vi "Begin.vi"(8 "error in":errorcluster) -> (0 "error out":errorcluster)   [LabVIEW 2016]
doc: "Called before other user functions, this VI is expected to open initial I/O refnums, load in file data, and do all program initialization. Notice that the <B>error out</B> terminal is simply used for data flow. Wiring it to other structures or subVIs ensures that this VI runs first."
uses:
  <vilib>/Rock Robotics/WPI/DriverStation/WPI_DriverStationRobotMode2.ctl
  Control Files/DriveMotors.ctl
  Control Files/Extra Motors.ctl
  <vilib>/Rock Robotics/WPI/ThirdParty/CanMotor/TalonSRX/WPI_CANTalonSRX_APIControlMode.ctl
  Control Files/Controllers.ctl
  <vilib>/Rock Robotics/WPI/Joystick/WPI_JoystickDeviceEnum.ctl
  <vilib>/Rock Robotics/WPI/SafetyOutput/WPI_SafetyOutputConfigMenu.ctl
  Control Files/SwerveMotors.ctl
  <vilib>/Rock Robotics/WPI/ThirdParty/CanMotor/TalonSRX/WPI_CANTalonSRX_APIFeedbackSelect.ctl
  Robot Global Data.vi
panel:
  in  "PID gains":T1={"proportional gain (Kc)"=5.0, "integral time (Ti, min)"=0.032, "derivative time (Td, min)"=0.0} {"derivative time (Td, min)" format="%.3f"; "integral time (Ti, min)" format="%.8f"; "proportional gain (Kc)" format="%.8f"}
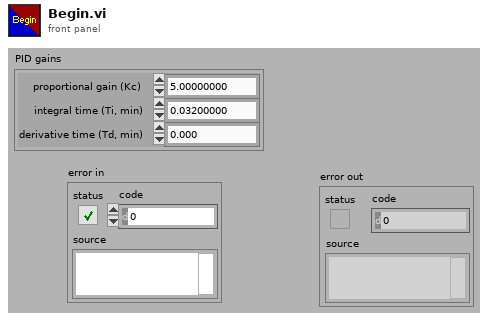
[diagram p1: front panel]
types:
  T1 = cluster{"proportional gain (Kc)":dbl, "integral time (Ti, min)":dbl, "derivative time (Td, min)":dbl}
  T2 = typedef "WPI_SafetyOutputConfigMenu.ctl" = enum16{"Enable", "Disable"}
  T3 = typedef "WPI_JoystickDeviceEnum.ctl" = enum16{"USB 0", "USB 1", "USB 2", "USB 3", "USB 4", "USB 5"}
  T4 = typedef "Controllers.ctl" = enum16{"Controller", "Controller2"}
  T5 = typedef "WPI_CANTalonSRX_APIControlMode.ctl" = enum8{"Percent VBus", "Speed", "Position", "Slave", "Unchanged / Invalid", "Voltage Compensation", "Current", "Motion Profile", "Motion Magic"}
  T6 = typedef "Extra Motors.ctl" = enum16{"Climber"}
  T7 = typedef "DriveMotors.ctl" = enum16{"Drive1", "Drive2", "Drive3", "Drive4"}
  T8 = typedef "WPI_DriverStationRobotMode2.ctl" = enum16{"Autonomous Disabled", "Autonomous Enabled", "Teleop Disabled", "Teleop Enabled", "Disconnected", "Finish", "Test Disabled", "Test Enabled", "Emergency Stopped"}
  T9 = typedef "WPI_CANTalonSRX_APIFeedbackSelect.ctl" = enum16{"Digital Quadrature Encoder", "Analog Potentiometer", "Analog Encoder", "Count on Quad-A (Rising-Edge)", "Count on Quad-A (Falling-Edge)", "CTR Magnetic Enc (Absolute)", "CTR Magnetic Enc (Relative)", "Pulse Width"}
  T10 = typedef "SwerveMotors.ctl" = enum16{"Swerve 1", "Swerve 2", "Swerve 3", "Swerve 4"}
  T11 = typedef "WPI_MotorControlDeviceRef.ctl" = cluster{"DeviceStatus":errorcluster, "Type":T12, "PWM":cluster{"PWM Channel":T13, "DeadBand":T14}, "CAN":cluster{"Device Number":u8, "SetOutput VI Ref":variant, "GetOutput VI Ref":variant, "Enable VI Ref":variant, "Disable VI Ref":variant, "Data":variant}, "Invert":bool}
  T12 = typedef "WPI_MotorControlType.ctl" = enum16{"PWM", "CAN"}
  T13 = typedef "FPGA_DIOPWMChannel.ctl" = enum8{"PWM 0", "PWM 1", "PWM 2", "PWM 3", "PWM 4", "PWM 5", "PWM 6", "PWM 7", "PWM 8", "PWM 9", "PWM MXP 0", "PWM MXP 1", "PWM MXP 2", "PWM MXP 3", "PWM MXP 4", "PWM MXP 5", "PWM MXP 6", "PWM MXP 7", "PWM MXP 8", "PWM MXP 9", "Invalid"}
  T14 = typedef "WPI_PWMDeadband.ctl" = cluster{"Name":string, "maxPositivePwm":i32, "minPositivePwm":i32, "centerPwm":i32, "maxNegativePwm":i32, "minNegativePwm":i32, "angularRange":u16}
  T15 = typedef "WPI_JoystickDevRef.ctl" = cluster{"Device":T3}
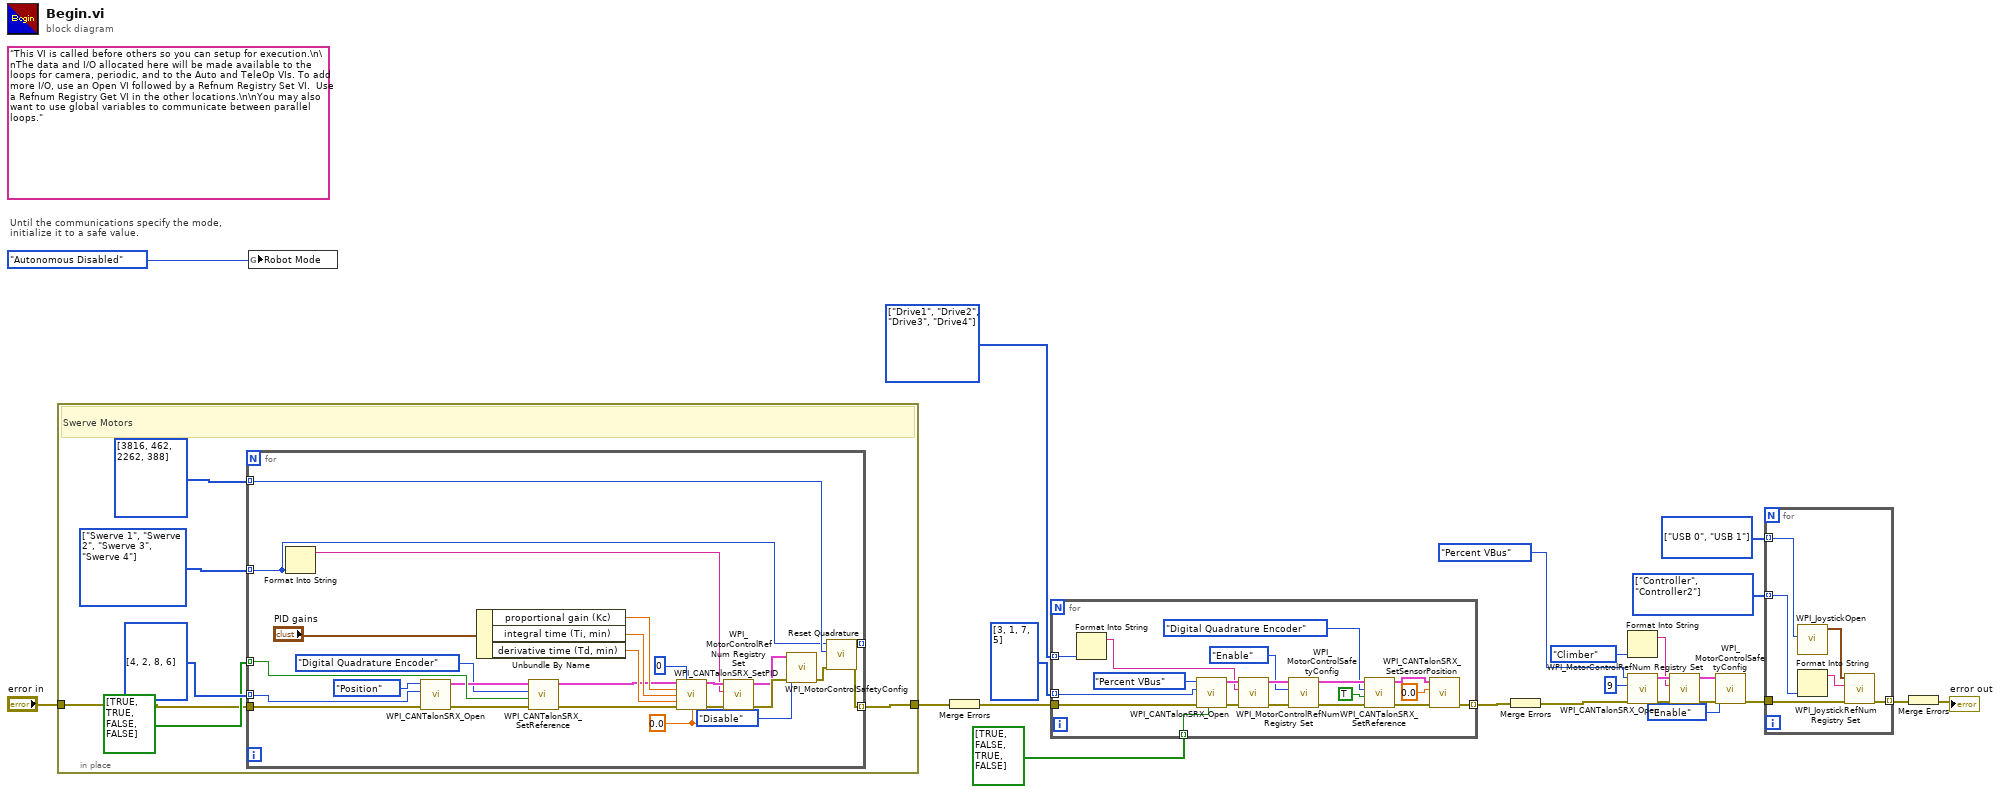
[diagram p0: block diagram]
diagram:
  w6 = T3[] [enum."USB 0", enum."USB 1"] items=["USB 0", "USB 1", "USB 2", "USB 3", "USB 4", "USB 5"] ("Array")
  w7 = T4[] [enum."Controller", enum."Controller2"] items=["Controller", "Controller2"] ("Array")
  w20 = T7[] [enum."Drive1", enum."Drive2", enum."Drive3", enum."Drive4"] items=["Drive1", "Drive2", "Drive3", "Drive4"]
  (unwired) "This VI is called before others so you can setup for execution.\n\nThe data and I/O allocated here will be made available to the loops for camera, periodic, and to the Auto and TeleOp VIs. To add more I/O, use an Open VI followed by a Refnum Registry Set VI.  Use a Refnum Registry Get VI in the other locations.\n\nYou may also want to use global variables to communicate between parallel loops."
  # "Until the communications specify the mode,\ninitialize it to a safe value."
  n1 = in-place {
    in-place-border: "error in" -> [w26]
    in-place-border: [w24] -> w21
    w29 = T10[] [enum."Swerve 1", enum."Swerve 2", enum."Swerve 3", enum."Swerve 4"] items=["Swerve 1", "Swerve 2", "Swerve 3", "Swerve 4"]
    # "Swerve Motors"
    n2 = for {
      tunnel: w29 -> [w33] mode=indexing
      tunnel: u8[] [4, 2, 8, 6] -> [w51] mode=indexing
      tunnel: w26 -> [w49]
      tunnel: bool[] [TRUE, TRUE, FALSE, FALSE] -> [w40] mode=indexing
      tunnel: i32[] [3816, 462, 2262, 388] -> [w34] mode=indexing
      tunnel: [w31] -> w24 mode=indexing
      tunnel: [w30] -> _ mode=indexing
      w41 = 0.0
      n3 = Format Into String(w33) -> (resulting string=w46:string)  [unwired: 3 in, 1 out]
      n4 = call <vilib>:"WPI_CANTalonSRX_Open.vi"("error in"=w49, "Device Number"=w51, "Control Mode"=WPI_CANTalonSRX_APIControlMode."Position") -> ("error out"=w54:errorcluster, "CAN Talon SRX Ref"=w39:T11)  [unwired: 7 in]
      n5 = Unbundle By Name("PID gains") -> ("proportional gain (Kc)"=w44:dbl, "integral time (Ti, min)"=w43:dbl, "derivative time (Td, min)"=w42:dbl)
      n6 = call <vilib>:"WPI_CANTalonSRX_SetReference.vi"("error in (no error)"=w54, "Reverse Feedback Sensor"=w40, "Feedback Reference"=WPI_CANTalonSRX_APIFeedbackSelect."Digital Quadrature Encoder", "CAN Talon SRX Ref"=w39) -> ("error out"=w53:errorcluster, "CAN Talon SRX Ref"=w38:T11)  [unwired: 6 in]
      n7 = call <vilib>:"WPI_CANTalonSRX_SetPID.vi"("CAN Talon SRX Ref"=w38, "Parameter Slot"=u8 0, "P"=w44, "I"=w43, "D"=w42, "error in (no error)"=w53, "I Zone"=w41, "Ramp Rate"=w41) -> ("CAN Talon SRX Ref"=w47:T11, "error out"=w52:errorcluster)  [unwired: 6 in]
      n8 = call <vilib>:"WPI_MotorControlRefNum Registry Set.vi"("error in (no error)"=w52, "refnum name"=w46, "MotorControlDevRef"=w47) -> ("error out"=w55:errorcluster, "MotorControlDevRef"=w48:T11)  [unwired: 7 in]
      n9 = call <vilib>:"WPI_MotorControlSafetyConfig.vi"("error in (no error)"=w55, "mode"=WPI_SafetyOutputConfigMenu."Disable", "MotorControlDevRef"=w48) -> ("error out"=w32:errorcluster)  [unwired: 7 in, 1 out]
      n10 = call "Reset Quadrature.vi"("error in"=w32, "Forward Position"=w34, "Enum"=w33) -> ("error out"=w31:errorcluster, "Encoder Offset"=w30:i32)  [unwired: 7 in]
    }
  }
  n11 = global write "Robot Global Data.vi" "Robot Mode"(WPI_DriverStationRobotMode2."Autonomous Disabled" ("Robot Mode")) -> ()
  n12 = Merge Errors(w21) -> (w18:errorcluster)
  n13 = for {
    tunnel: w20 -> [w74] mode=indexing
    tunnel: i32[] [3, 1, 7, 5] -> [w73] mode=indexing
    tunnel: w18 -> [w58]
    tunnel: [w57] -> w17 mode=indexing
    tunnel: bool[] [TRUE, FALSE, TRUE, FALSE] -> [w56] mode=indexing
    n14 = Format Into String(w74) -> (resulting string=w70:string)  [unwired: 3 in, 1 out]
    n15 = call <vilib>:"WPI_CANTalonSRX_Open.vi"("Invert"=w56, "error in"=w58, "Device Number"=w73, "Control Mode"=WPI_CANTalonSRX_APIControlMode."Percent VBus") -> ("error out"=w72:errorcluster, "CAN Talon SRX Ref"=w71:T11)  [unwired: 6 in]
    n16 = call <vilib>:"WPI_MotorControlRefNum Registry Set.vi"("error in (no error)"=w72, "refnum name"=w70, "MotorControlDevRef"=w71) -> ("error out"=w68:errorcluster, "MotorControlDevRef"=w67:T11)  [unwired: 7 in]
    n17 = call <vilib>:"WPI_MotorControlSafetyConfig.vi"("error in (no error)"=w68, "mode"=WPI_SafetyOutputConfigMenu."Enable", "MotorControlDevRef"=w67) -> ("error out"=w65:errorcluster, "MotorControlDevRef"=w64:T11)  [unwired: 7 in]
    n18 = call <vilib>:"WPI_CANTalonSRX_SetReference.vi"("error in (no error)"=w65, "Reverse Feedback Sensor"=TRUE, "Feedback Reference"=WPI_CANTalonSRX_APIFeedbackSelect."Digital Quadrature Encoder", "CAN Talon SRX Ref"=w64) -> ("error out"=w60:errorcluster, "CAN Talon SRX Ref"=w61:T11)  [unwired: 6 in]
    n19 = call <vilib>:"WPI_CANTalonSRX_SetSensorPosition.vi"("error in (no error)"=w60, "New Sensor Position"=0.0, "CAN Talon SRX Ref"=w61) -> ("error out"=w57:errorcluster)  [unwired: 7 in, 1 out]
  }
  n20 = Merge Errors(w17) -> (w12:errorcluster)
  n21 = Format Into String(Extra_Motors."Climber") -> (resulting string=w10:string)  [unwired: 3 in, 1 out]
  n22 = call <vilib>:"WPI_CANTalonSRX_Open.vi"("error in"=w12, "Device Number"=u8 9, "Control Mode"=WPI_CANTalonSRX_APIControlMode."Percent VBus") -> ("error out"=w16:errorcluster, "CAN Talon SRX Ref"=w15:T11)  [unwired: 7 in]
  n23 = call <vilib>:"WPI_MotorControlRefNum Registry Set.vi"("error in (no error)"=w16, "refnum name"=w10, "MotorControlDevRef"=w15) -> ("error out"=w14:errorcluster, "MotorControlDevRef"=w13:T11)  [unwired: 7 in]
  n24 = call <vilib>:"WPI_MotorControlSafetyConfig.vi"("error in (no error)"=w14, "mode"=WPI_SafetyOutputConfigMenu."Enable", "MotorControlDevRef"=w13) -> ("error out"=w5:errorcluster)  [unwired: 7 in, 1 out]
  n25 = for {
    tunnel: w7 -> [w80] mode=indexing
    tunnel: w6 -> [w78] mode=indexing
    tunnel: w5 -> [w76]
    tunnel: [w75] -> w4 mode=indexing
    n26 = call <vilib>:"WPI_JoystickOpen.vi"("JoystickDevice"=w78) -> ("JoystickDevRef"=w77:T15)  [unwired: 10 in]
    n27 = Format Into String(w80) -> (resulting string=w79:string)  [unwired: 3 in, 1 out]
    n28 = call <vilib>:"WPI_JoystickRefNum Registry Set.vi"("error in (no error)"=w76, "refnum name"=w79, "JoystickDevRef"=w77) -> ("error out"=w75:errorcluster)  [unwired: 7 in, 1 out]
  }
  n29 = Merge Errors(w4) -> (→"error out":errorcluster)
